vi "motorEncAngleVelocity.vi"(8 "dt":dbl=0.001 format="%#_13g", 9 "CPR":dbl=2048.0 format="%#_13g", 10 "error in (no error)":errorcluster, 11 "Refnum in":refnum<k20>) -> (0 "error out":errorcluster, 1 "CableReelPos(deg)":dbl[](array[numeric]), 2 "Refnum out":refnum<k20>, 3 "CableReelVel(RPM)":dbl[](array[numeric]))   [LabVIEW 2017]
uses:
  <vilib>/rvi/interface/nirviReadWriteControl/nirviReadWriteControl.xnode
  NiFpgaLv.dll
  <vilib>/Utility/error.llb/Error Cluster From Error Code.vi
  <vilib>/rvi/interface/Simulation/niFpgaSimulationCallBeginRW.vi
  <vilib>/rvi/errors/niLvFpgaAdjustHostInterfaceError.vi
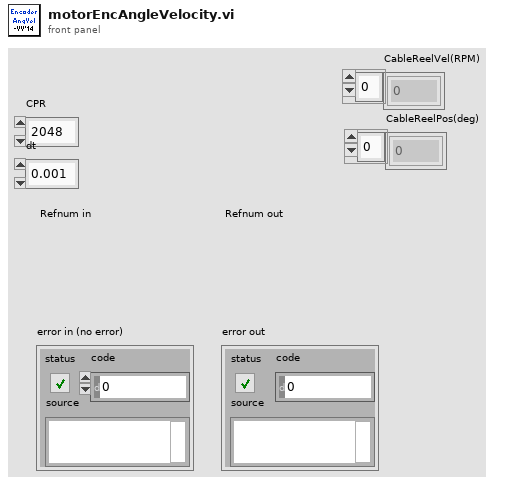
[diagram p1: front panel]
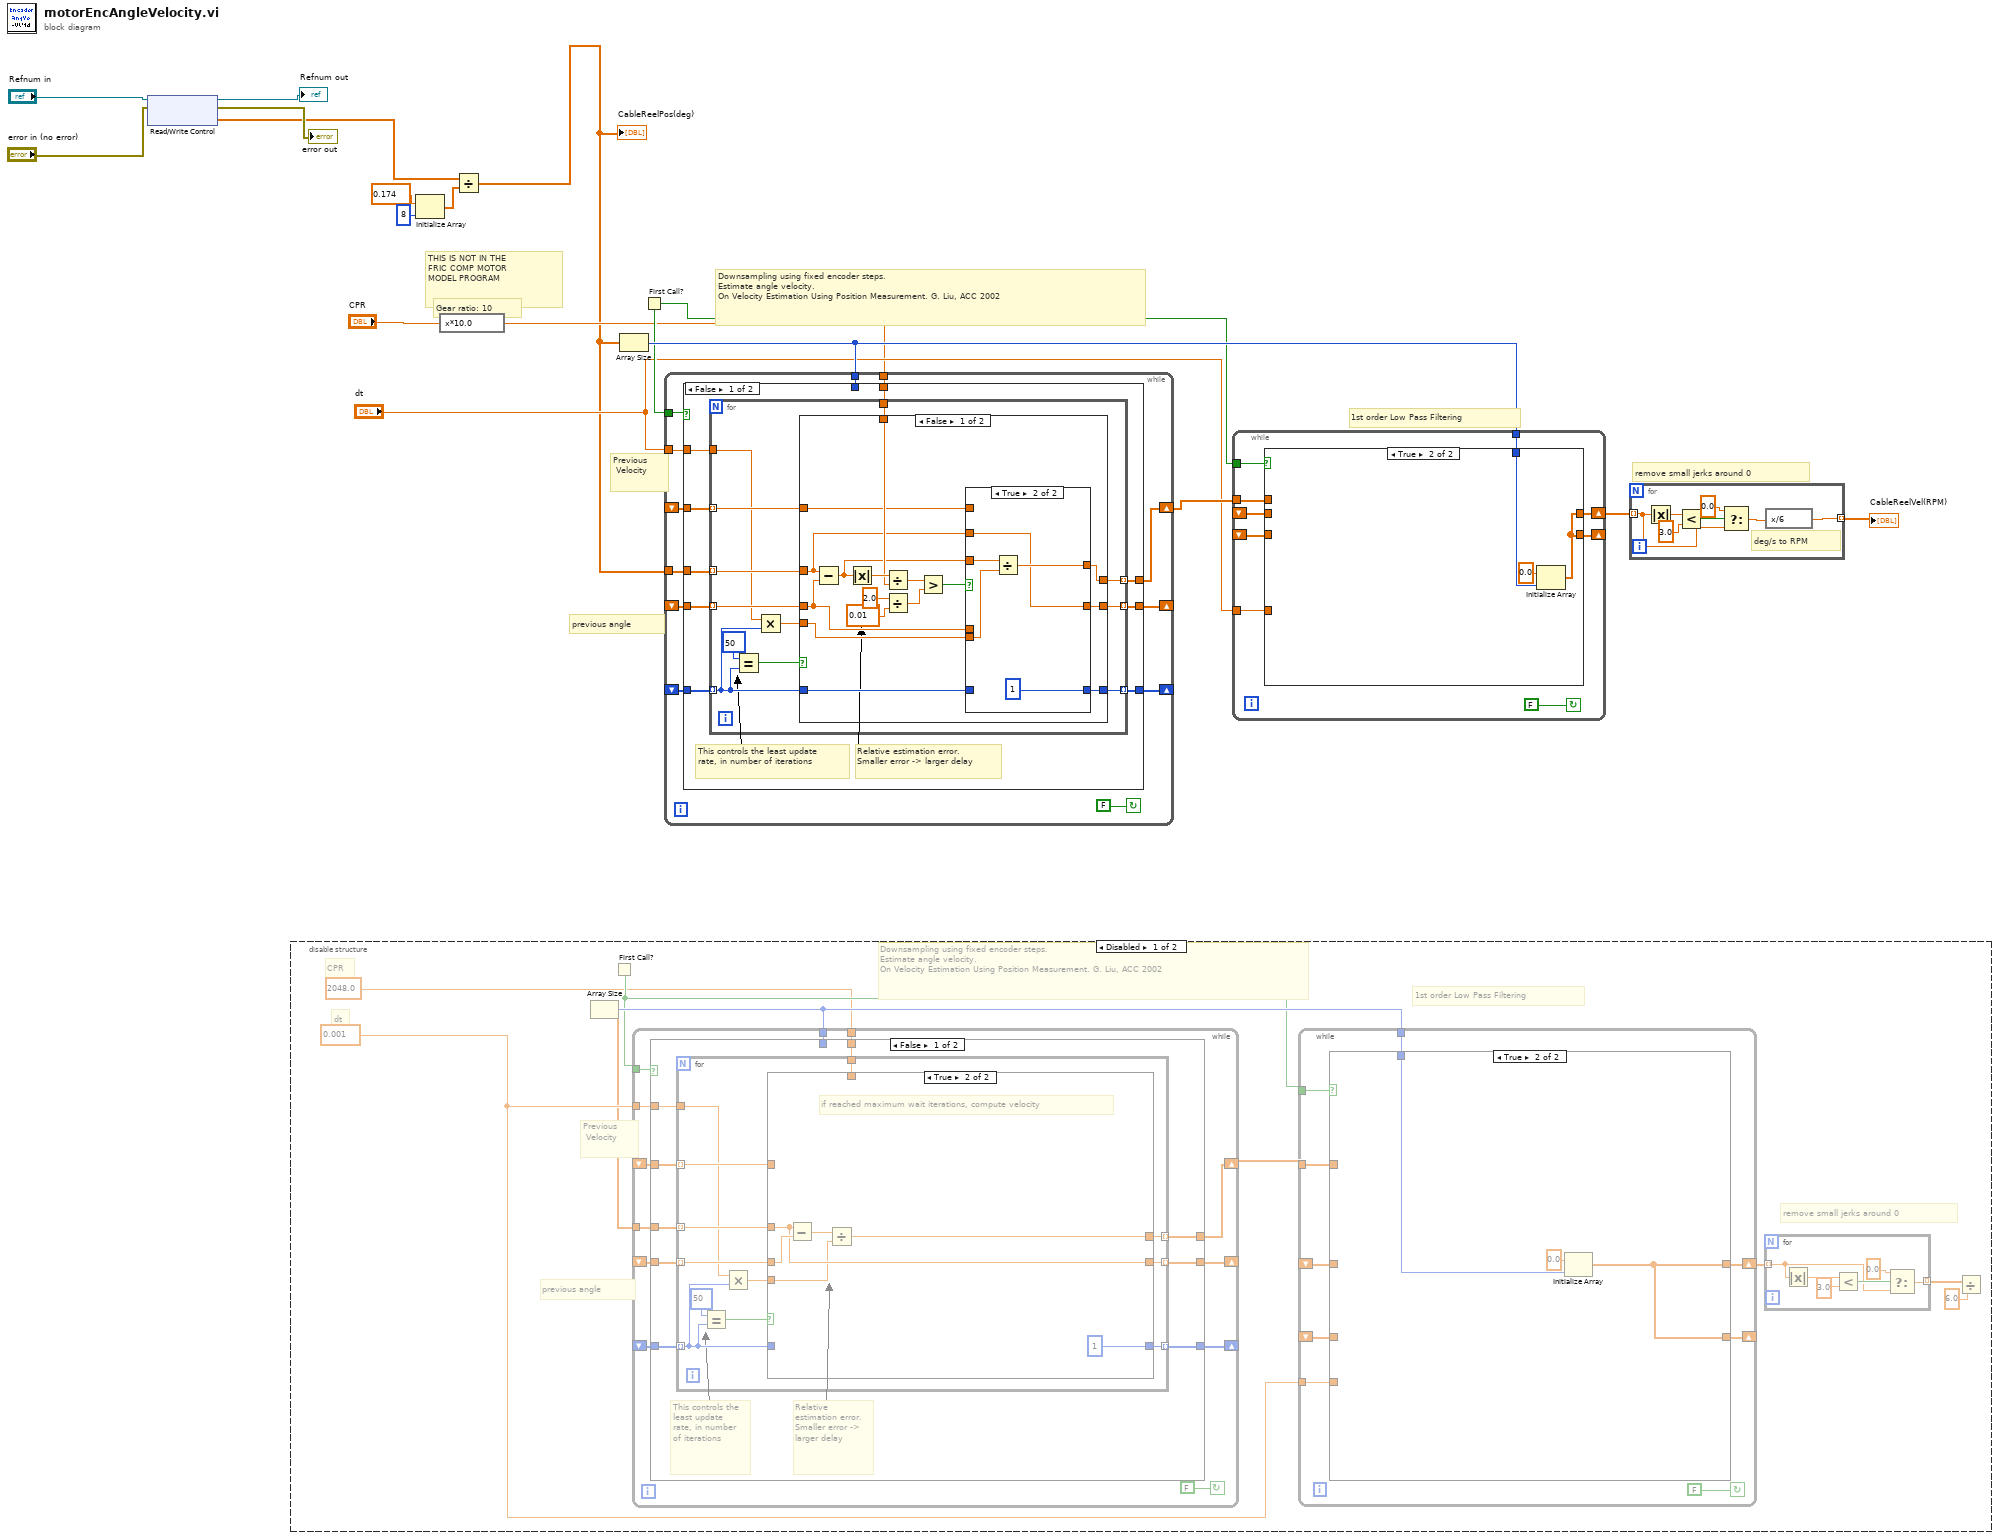
[diagram p0: block diagram]
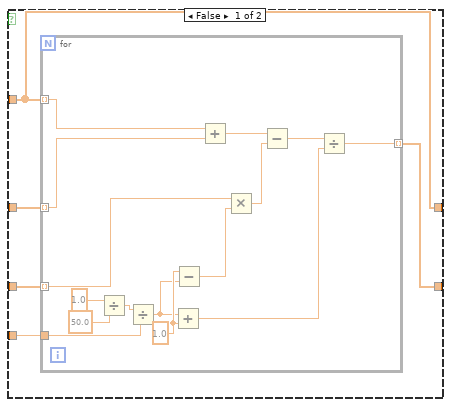
[diagram p2: hidden frame]
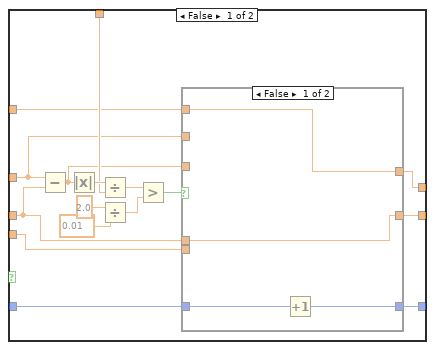
[diagram p3: hidden frame]
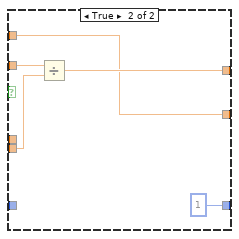
[diagram p4: hidden frame]
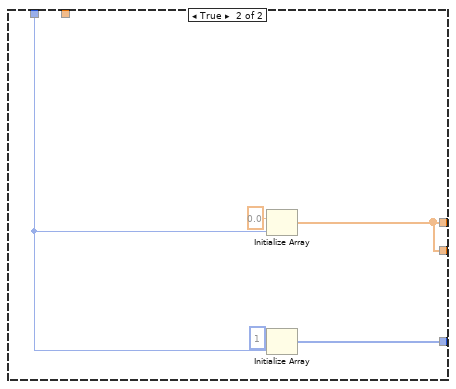
[diagram p5: hidden frame]
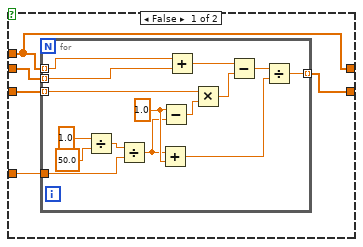
[diagram p7: hidden frame]
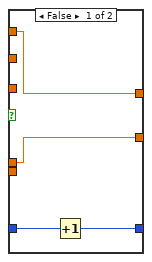
[diagram p8: hidden frame]
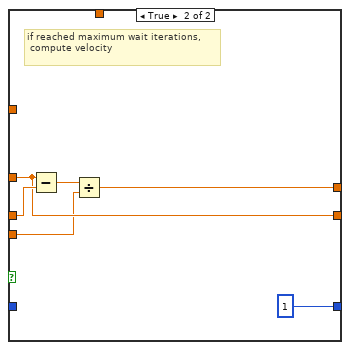
[diagram p9: hidden frame]
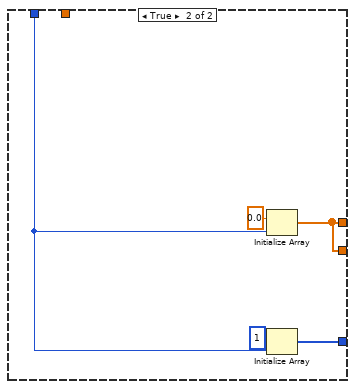
[diagram p10: hidden frame]
diagram:
  # "THIS IS NOT IN THE\nFRIC COMP MOTOR \nMODEL PROGRAM"
  # "Gear ratio: 10"
  # "remove small jerks around 0"
  # "Downsampling using fixed encoder steps.\nEstimate angle velocity. \nOn Velocity Estimation Using Position Measurement. G. Liu, ACC 2002"
  # "1st order Low Pass Filtering"
  # "Previous\n Velocity"
  # "previous angle"
  n1 = xnode "Read/Write Control"("FPGA VI Reference In"="Refnum in", "error in"="error in (no error)") -> ("FPGA VI Reference Out"=→"Refnum out":refnum<k20>, "error out"=→"error out":errorcluster, "EncdAngle"=w2:sgl[])
  n2 = disable-structure shown="Disabled" {
    frame Disabled {
      w22 = 0.001
      # "dt"
      # "CPR"
      # "remove small jerks around 0"
      # "Downsampling using fixed encoder steps.\nEstimate angle velocity. \nOn Velocity Estimation Using Position Measurement. G. Liu, ACC 2002"
      # "1st order Low Pass Filtering"
      # "Previous\n Velocity"
      # "previous angle"
      n3 = First Call?() -> (First Call?: T/F=w24:bool)
      n4 = Array Size(array=w18) -> (size(s)=w25:i32)
      n5 = while {
        tunnel: [w76] -> w18
        shift-right: [w73] -> _
        shift-left: _ -> [w74]
        shift-right: [w70] -> _
        shift-left: _ -> [w72]
        shift-right: [w71] -> w26
        shift-left: _ -> [w68]
        tunnel: 2048.0 -> [w69]
        tunnel: w22 -> [w67]
        tunnel: w24 -> [w66]
        tunnel: w25 -> [w65]
        stop <- FALSE continue-if-true
        n6 = case shown="False" w66 {
          tunnel: w76 -> [w85 _]
          tunnel: w74 -> [w84 _]
          tunnel: [w83 w131] -> w73
          tunnel: w72 -> [w82 _]
          tunnel: [w81 w130] -> w71
          tunnel: [w80 w130] -> w70
          tunnel: w69 -> [w79 _]
          tunnel: w68 -> [w78 _]
          tunnel: w67 -> [w77 _]
          tunnel: w65 -> [_ w129]
          frame False {
            # "Relative estimation error. Smaller error -> larger delay"
            # "This controls the least update rate, in number of iterations"
            n7 = for {
              tunnel: w85 -> [w94] mode=indexing
              tunnel: [w95] -> w83 mode=indexing
              tunnel: w84 -> [w87] mode=indexing
              tunnel: w82 -> [w93] mode=indexing
              tunnel: [w92] -> w81 mode=indexing
              tunnel: [w91] -> w80 mode=indexing
              tunnel: w79 -> [w90]
              tunnel: w78 -> [w88] mode=indexing
              tunnel: w77 -> [w86]
              n8 = Equal?(x=50, y=w87) -> (x = y?=w96:bool)
              n9 = Multiply(x=w86, y=w87) -> (x*y=w89:dbl)
              n10 = case shown="True" w96 {
                tunnel: [w101 1 ("sample length")] -> w95
                tunnel: w89 -> [w106 w123]
                tunnel: w94 -> [w103 w124]
                tunnel: w93 -> [w100 w127]
                tunnel: [w104 w125] -> w92
                tunnel: [w102 w124] -> w91
                tunnel: w90 -> [w112 _]
                tunnel: w88 -> [w99 _]
                tunnel: w87 -> [w98 _]
                frame False {
                  n11 = Subtract(x=w103, y=w100) -> (x-y=w105:dbl)
                  n12 = Absolute Value(x=w105) -> (abs(x)=w113:dbl)
                  n13 = Divide(x=w113, y=w112) -> (x/y=w111:dbl)
                  n14 = Divide(x=2.0, y=0.01) -> (x/y=w108:dbl)
                  n15 = Greater?(x=w111, y=w108) -> (0:w107:bool)
                  n16 = case shown="False" w107 {
                    tunnel: w106 -> [_ w121]
                    tunnel: w105 -> [_ w122]
                    tunnel: [w116 w120] -> w104
                    tunnel: w103 -> [_ w119]
                    tunnel: [w117 w119] -> w102
                    tunnel: [w114 1 ("sample length")] -> w101
                    tunnel: w100 -> [w117 _]
                    tunnel: w99 -> [w116 _]
                    tunnel: w98 -> [w115 _]
                    frame False {
                      n17 = Increment(x=w115) -> (x+1=w114:i32)
                    }
                    frame True {
                      n18 = Divide(x=w122, y=w121) -> (x/y=w120:dbl)
                    }
                  }
                }
                frame True {
                  # "if reached maximum wait iterations, compute velocity"
                  n19 = Subtract(x=w124, y=w127) -> (x-y=w126:dbl)
                  n20 = Divide(x=w126, y=w123) -> (x/y=w125:dbl)
                }
              }
            }
          }
          frame True {
            n21 = Initialize Array(0.0, w129) -> (w130:dbl[])
            n22 = Initialize Array(1 ("sample length"), w129) -> (w131:i32[])
          }
        }
      }
      n23 = while {
        tunnel: w22 -> [w34]
        shift-right: [w38] -> w23
        shift-left: _ -> [w36]
        shift-right: [w37] -> _
        shift-left: _ -> [w35]
        tunnel: w26 -> [w41]
        tunnel: w24 -> [w40]
        tunnel: w25 -> [w39]
        stop <- FALSE continue-if-true
        n24 = case shown="True" w40 {
          tunnel: w41 -> [w42 _]
          tunnel: w39 -> [_ w63]
          tunnel: [w42 w62] -> w38
          tunnel: [w43 w62] -> w37
          tunnel: w36 -> [w46 _]
          tunnel: w35 -> [w45 _]
          tunnel: w34 -> [w44 _]
          frame False {
            n25 = for {
              tunnel: w42 -> [w54] mode=indexing
              tunnel: w46 -> [w53] mode=indexing
              tunnel: w45 -> [w52] mode=indexing
              tunnel: w44 -> [w51]
              tunnel: [w47] -> w43 mode=indexing
              w60 = 1.0 ("y")
              n26 = Divide(x=1.0, y=50.0) -> (x/y=w48:dbl)
              n27 = Divide(x=w48, y=w51) -> (x/y=w59:dbl)
              n28 = Add(x=w59, y=w60) -> (x+y=w57:dbl)
              n29 = Subtract(x=w60, y=w59) -> (x-y=w56:dbl)
              n30 = Add(x=w54, y=w53) -> (x+y=w61:dbl)
              n31 = Multiply(x=w52, y=w56) -> (x*y=w55:dbl)
              n32 = Subtract(x=w61, y=w55) -> (x-y=w58:dbl)
              n33 = Divide(x=w58, y=w57) -> (x/y=w47:dbl)
            }
          }
          frame True {
            n34 = Initialize Array(0.0, w63) -> (w62:dbl[])
          }
        }
      }
      n35 = for {
        tunnel: w23 -> [w28] mode=indexing
        tunnel: [w27] -> w19 mode=indexing
        n36 = Absolute Value(x=w28) -> (abs(x)=w32:dbl)
        n37 = Less?(x=w32, y=3.0) -> (x < y?=w30:bool)
        n38 = Select(t=0.0, s=w30, f=w28) -> (s? t:f=w27:dbl)
      }
      n39 = Divide(x=w19, y=6.0) -> ()  [unwired: 1 out]
    }
    frame Enabled {
    }
  }
  n40 = Initialize Array(0.174 ("element"), 8 ("dimension size")) -> (w3:dbl[])
  n41 = expression code="x*10.0"("CPR") -> (w10:dbl)
  n42 = Divide(x=w2, y=w3) -> (x/y=w1:dbl[])
  "CableReelPos(deg)" <- w1
  n43 = Array Size(array=w1) -> (size(s)=w16:i32)
  n44 = First Call?() -> (First Call?: T/F=w15:bool)
  n45 = while {
    tunnel: w1 -> [w145]
    shift-right: [w142] -> _
    shift-left: _ -> [w143]
    shift-right: [w139] -> _
    shift-left: _ -> [w141]
    shift-right: [w140] -> w17
    shift-left: _ -> [w137]
    tunnel: w10 -> [w138]
    tunnel: "dt" -> [w136]
    tunnel: w15 -> [w135]
    tunnel: w16 -> [w134]
    stop <- FALSE continue-if-true
    n46 = case shown="False" w135 {
      tunnel: w145 -> [w154 _]
      tunnel: w143 -> [w153 _]
      tunnel: [w152 w200] -> w142
      tunnel: w141 -> [w151 _]
      tunnel: [w150 w199] -> w140
      tunnel: [w149 w199] -> w139
      tunnel: w138 -> [w148 _]
      tunnel: w137 -> [w147 _]
      tunnel: w136 -> [w146 _]
      tunnel: w134 -> [_ w198]
      frame False {
        # "Relative estimation error. Smaller error -> larger delay"
        # "This controls the least update rate, in number of iterations"
        n47 = for {
          tunnel: w154 -> [w163] mode=indexing
          tunnel: [w164] -> w152 mode=indexing
          tunnel: w153 -> [w156] mode=indexing
          tunnel: w151 -> [w162] mode=indexing
          tunnel: [w161] -> w150 mode=indexing
          tunnel: [w160] -> w149 mode=indexing
          tunnel: w148 -> [w159]
          tunnel: w147 -> [w157] mode=indexing
          tunnel: w146 -> [w155]
          n48 = Equal?(x=50, y=w156) -> (x = y?=w165:bool)
          n49 = Multiply(x=w155, y=w156) -> (x*y=w158:dbl)
          n50 = case shown="False" w165 {
            tunnel: [w170 1 ("sample length")] -> w164
            tunnel: w158 -> [w175 w192]
            tunnel: w163 -> [w172 w193]
            tunnel: w162 -> [w169 w196]
            tunnel: [w173 w194] -> w161
            tunnel: [w171 w193] -> w160
            tunnel: w159 -> [w181 _]
            tunnel: w157 -> [w168 _]
            tunnel: w156 -> [w167 _]
            frame False {
              n51 = Subtract(x=w172, y=w169) -> (x-y=w174:dbl)
              n52 = Absolute Value(x=w174) -> (abs(x)=w182:dbl)
              n53 = Divide(x=w182, y=w181) -> (x/y=w180:dbl)
              n54 = Divide(x=2.0, y=0.01) -> (x/y=w177:dbl)
              n55 = Greater?(x=w180, y=w177) -> (0:w176:bool)
              n56 = case shown="True" w176 {
                tunnel: w175 -> [_ w190]
                tunnel: w174 -> [_ w191]
                tunnel: [w185 w189] -> w173
                tunnel: w172 -> [_ w188]
                tunnel: [w186 w188] -> w171
                tunnel: [w183 1 ("sample length")] -> w170
                tunnel: w169 -> [w186 _]
                tunnel: w168 -> [w185 _]
                tunnel: w167 -> [w184 _]
                frame False {
                  n57 = Increment(x=w184) -> (x+1=w183:i32)
                }
                frame True {
                  n58 = Divide(x=w191, y=w190) -> (x/y=w189:dbl)
                }
              }
            }
            frame True {
              # "if reached maximum wait iterations,\n compute velocity"
              n59 = Subtract(x=w193, y=w196) -> (x-y=w195:dbl)
              n60 = Divide(x=w195, y=w192) -> (x/y=w194:dbl)
            }
          }
        }
      }
      frame True {
        n61 = Initialize Array(0.0, w198) -> (w199:dbl[])
        n62 = Initialize Array(1 ("sample length"), w198) -> (w200:i32[])
      }
    }
  }
  n63 = while {
    tunnel: "dt" -> [w204]
    shift-right: [w208] -> w14
    shift-left: _ -> [w206]
    shift-right: [w207] -> _
    shift-left: _ -> [w205]
    tunnel: w17 -> [w211]
    tunnel: w15 -> [w210]
    tunnel: w16 -> [w209]
    stop <- FALSE continue-if-true
    n64 = case shown="True" w210 {
      tunnel: w211 -> [w212 _]
      tunnel: w209 -> [_ w233]
      tunnel: [w212 w232] -> w208
      tunnel: [w213 w232] -> w207
      tunnel: w206 -> [w216 _]
      tunnel: w205 -> [w215 _]
      tunnel: w204 -> [w214 _]
      frame False {
        n65 = for {
          tunnel: w212 -> [w224] mode=indexing
          tunnel: w216 -> [w223] mode=indexing
          tunnel: w215 -> [w222] mode=indexing
          tunnel: w214 -> [w221]
          tunnel: [w217] -> w213 mode=indexing
          w230 = 1.0 ("y")
          n66 = Divide(x=1.0, y=50.0) -> (x/y=w218:dbl)
          n67 = Divide(x=w218, y=w221) -> (x/y=w229:dbl)
          n68 = Add(x=w229, y=w230) -> (x+y=w227:dbl)
          n69 = Subtract(x=w230, y=w229) -> (x-y=w226:dbl)
          n70 = Add(x=w224, y=w223) -> (x+y=w231:dbl)
          n71 = Multiply(x=w222, y=w226) -> (x*y=w225:dbl)
          n72 = Subtract(x=w231, y=w225) -> (x-y=w228:dbl)
          n73 = Divide(x=w228, y=w227) -> (x/y=w217:dbl)
        }
      }
      frame True {
        n74 = Initialize Array(0.0, w233) -> (w232:dbl[])
      }
    }
  }
  n75 = for {
    tunnel: w14 -> [w237] mode=indexing
    tunnel: [w236] -> w13 mode=indexing
    # "deg/s to RPM"
    n76 = Absolute Value(x=w237) -> (abs(x)=w241:dbl)
    n77 = Less?(x=w241, y=3.0) -> (x < y?=w239:bool)
    n78 = Select(t=0.0, s=w239, f=w237) -> (s? t:f=w235:dbl)
    n79 = expression code="x/6"(w235) -> (w236:dbl)
  }
  "CableReelVel(RPM)" <- w13
